vi "LabVIEW Coordinates to Picture Coordinates.vi"(8 "error in":errorcluster, 10 "CtlRef":refnum<vi>, 11 "LabVIEW Coordinates":cluster{"Horizontal":i32, "Vertical":i32}) -> (0 "error out":errorcluster, 3 "Picture Control Coordinates":cluster{"Horizontal":i32, "Vertical":i32})   [LabVIEW 2012, in "paint Xcontrol.xctl"]
uses:
  paint Xcontrol.xctl
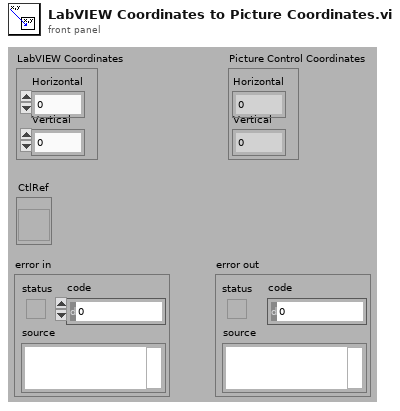
[diagram p1: front panel]
types:
  T1 = typedef "LVBoundsTypeDef.ctl" = cluster{"Width":u32, "Height":u32}
  T2 = typedef "LVPositionTypeDef.ctl" = cluster{"Left":i32, "Top":i32}
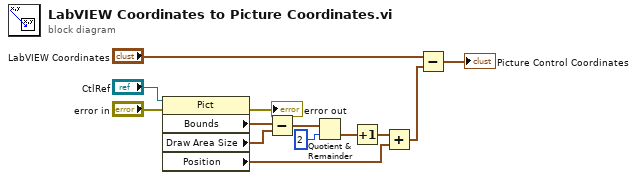
[diagram p0: block diagram]
diagram:
  n1 = property class="Pict"(reference="CtlRef", error in="error in") -> (error out=→"error out":errorcluster, "Bounds"=w7:T1, "Draw Area Size"=w2:T1, "Position"=w5:T2)  [unwired: 1 out]
  n2 = Subtract(x=w7, y=w2) -> (x-y=w9:T1)
  n3 = Quotient & Remainder(x=w9, y=u32 2) -> (floor(x/y)=w10:T1)  [unwired: 1 out]
  n4 = Increment(x=w10) -> (x+1=w1:T1)
  n5 = Add(x=w1, y=w5) -> (x+y=w4:T1)
  n6 = Subtract(x="LabVIEW Coordinates", y=w4) -> (x-y=→"Picture Control Coordinates":T1)
